vi "Alarmas_Bool.vi"() -> ()   [LabVIEW 2020]
panel:
  out "Waveform Chart":dbl(graph)
  in  "Lmin":u32(slide) scale=0.0..100.0
  in  "Lmax":u32(slide) scale=0.0..100.0
  out "Texto 3":string
  out "Texto 2":string
  out "Texto 1":string
  out "Alarma 3":bool
  out "Alarma 2":bool
  out "Alarma 1":bool
  in  "Temp 3":dbl(slide) scale=0.0..100.0
  in  "Temp 2":dbl(slide) scale=0.0..100.0
  in  "Temp 1":dbl(slide) scale=0.0..100.0
  # "Indicador de Alarmas"
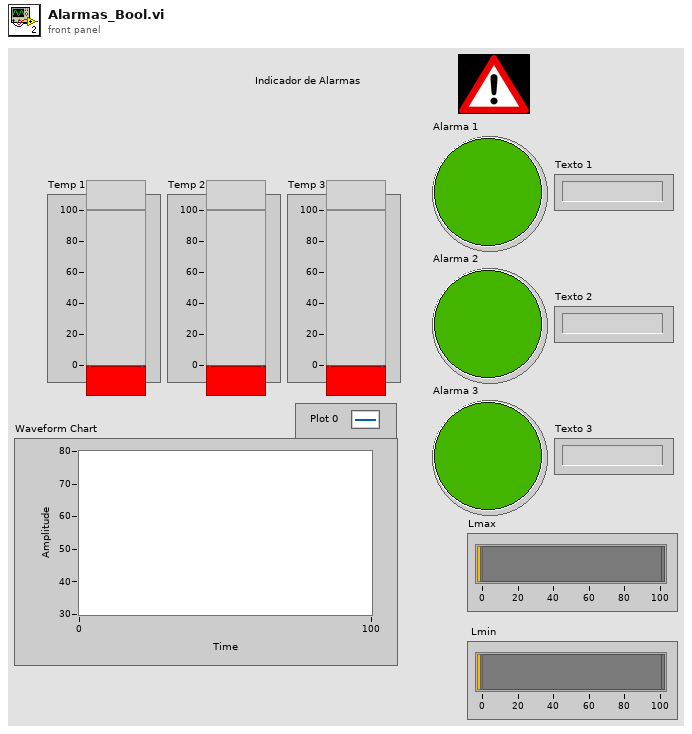
[diagram p1: front panel]
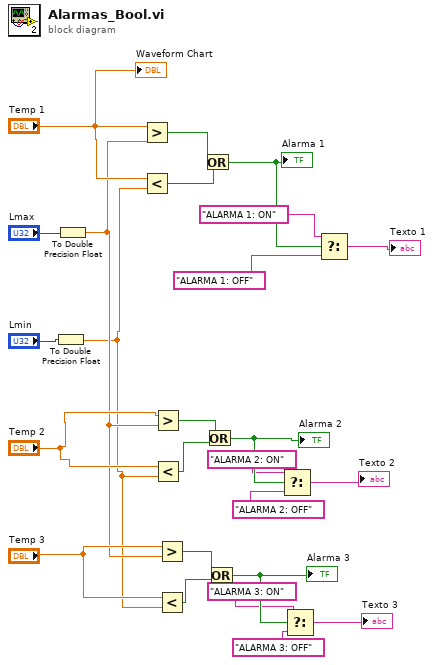
[diagram p0: block diagram]
diagram:
  n1 = To Double Precision Float(number="Lmin") -> (double precision float=w13:dbl)
  n2 = To Double Precision Float(number="Lmax") -> (double precision float=w14:dbl)
  n3 = Greater?(x="Temp 1", y=w14) -> (0:w21:bool)
  n4 = Less?(x="Temp 1", y=w13) -> (x < y?=w20:bool)
  n5 = Greater?(x="Temp 2", y=w14) -> (0:w19:bool)
  n6 = Less?(x="Temp 2", y=w13) -> (x < y?=w18:bool)
  n7 = Greater?(x="Temp 3", y=w14) -> (0:w17:bool)
  n8 = Less?(x="Temp 3", y=w13) -> (x < y?=w16:bool)
  n9 = Or(x=w21, y=w20) -> (x .or. y?=w12:bool)
  "Alarma 1" <- w12
  n10 = Or(x=w19, y=w18) -> (x .or. y?=w9:bool)
  "Alarma 2" <- w9
  n11 = Or(x=w17, y=w16) -> (x .or. y?=w6:bool)
  "Alarma 3" <- w6
  n12 = Select(t="ALARMA 2: ON", s=w9, f="ALARMA 2: OFF") -> (s? t:f=→"Texto 2":string)
  n13 = Select(t="ALARMA 3: ON", s=w6, f="ALARMA 3: OFF") -> (s? t:f=→"Texto 3":string)
  n14 = Select(t="ALARMA 1: ON", s=w12, f="ALARMA 1: OFF") -> (s? t:f=→"Texto 1":string)
  "Waveform Chart" <- "Temp 1"
